vi "CameraSetTrigger.vi"(8 "error in (no error)":errorcluster, 10 "external?":bool=TRUE, 11 "Photonfocus in":refnum<class "Photonfocus.lvclass">) -> (0 "error out":errorcluster, 2 "attribs":variant[](array[variant]), 3 "Photonfocus out":refnum<class "Photonfocus.lvclass">)   [LabVIEW 2010, in "Photonfocus.lvclass"]
uses:
  Photonfocus.lvclass
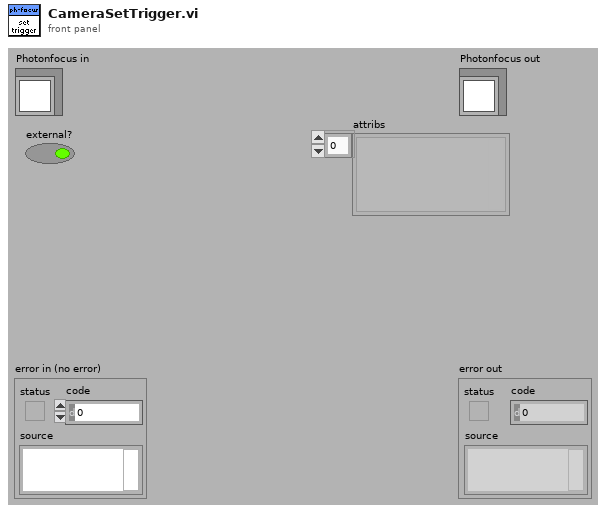
[diagram p1: front panel]
types:
  T1 = typedef "IMAQdx.ctl" = refnum<k21>
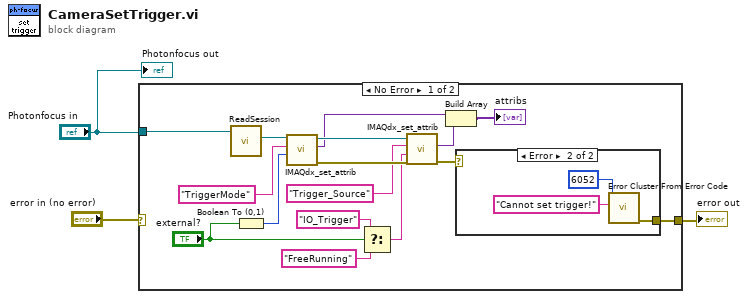
[diagram p0: block diagram]
diagram:
  n1 = case shown="No Error" "error in (no error)" {
    selector: "error in (no error)" -> [_ w23]
    tunnel: [w9 w23] -> w3
    tunnel: "Photonfocus in" -> [w5 _]
    frame No Error {
      n2 = call-dynamic "ReadSession.vi"("IMAQdx in"=w5) -> ("session"=w4:refnum<k21>)  [unwired: 9 in, 1 out]
      n3 = Boolean To (0,1)(Boolean="external?") -> (0, 1=w18:i16)
      n4 = call "IMAQdx_set_attrib.vi"("value"=w18, "attribute"="TriggerMode" ("ActiveAttribute"), "IMAQdx in"=w4) -> ("error out"=w16:errorcluster, "attrib out"=w6:variant, "IMAQdx out"=w17:T1)  [unwired: 2 in]
      n5 = Select(t="IO_Trigger" ("f"), s="external?", f="FreeRunning" ("attribute")) -> (s? t:f=w11:string)
      n6 = call "IMAQdx_set_attrib.vi"("error in"=w16, "value"=w11, "attribute"="Trigger_Source", "IMAQdx in"=w17) -> ("error out"=w10:errorcluster, "attrib out"=w7:variant)  [unwired: 1 in, 1 out]
      n7 = Build Array(w6, w7) -> (→"attribs":variant[])
      n8 = case shown="Error" w10 {
        tunnel: [_ w22] -> w9
        frame No Error {
        }
        frame Error {
          n9 = call <vilib>:"Error Cluster From Error Code.vi"("error message (\"\")"="Cannot set trigger!" ("error message (\"\")"), "error code (0)"=6052) -> ("error out"=w22:errorcluster)  [unwired: 7 in]
        }
      }
    }
    frame Error {
    }
  }
  "error out" <- w3
  "Photonfocus out" <- "Photonfocus in"
